vi "Add Coincident Event.vi"(8 "error in (no error)":errorcluster, 9 "Is Repeat Attempt":bool, 10 "Event":T1, 11 "Controller in":refnum<class "Controller.lvclass">) -> (0 "error out":errorcluster, 3 "Controller out":refnum<class "Controller.lvclass">)   [LabVIEW 2019, in "Controller.lvlib" / "Controller.lvclass"]
uses:
  Controller.lvclass
  <vilib>/ActorFramework/Actor/Actor.lvclass
  Controller Messages/New Event Msg/New Event Msg.lvclass
  C:/Program Files (x86)/National Instruments/LabVIEW 2019/vi.lib/ActorFramework/Actor/Actor.lvclass
  C:/Program Files (x86)/National Instruments/LabVIEW 2019/vi.lib/ActorFramework/Message/Message.lvclass
  Sensors/Detector/Event.ctl
  Sensors/Detector/Muon Detector.lvclass
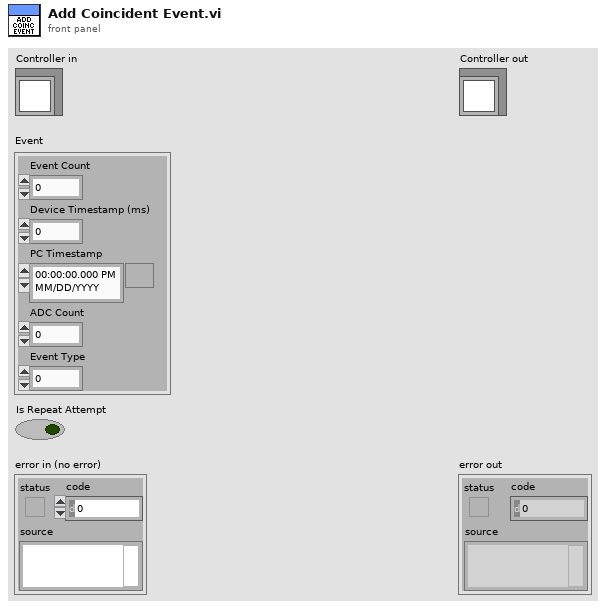
[diagram p1: front panel]
types:
  T1 = typedef "Muon Detector.lvclass/Event.ctl" = cluster{"Event Count":i32, "Device Timestamp (ms)":i32, "PC Timestamp":timestamp, "ADC Count":i32, "Event Type":u8}
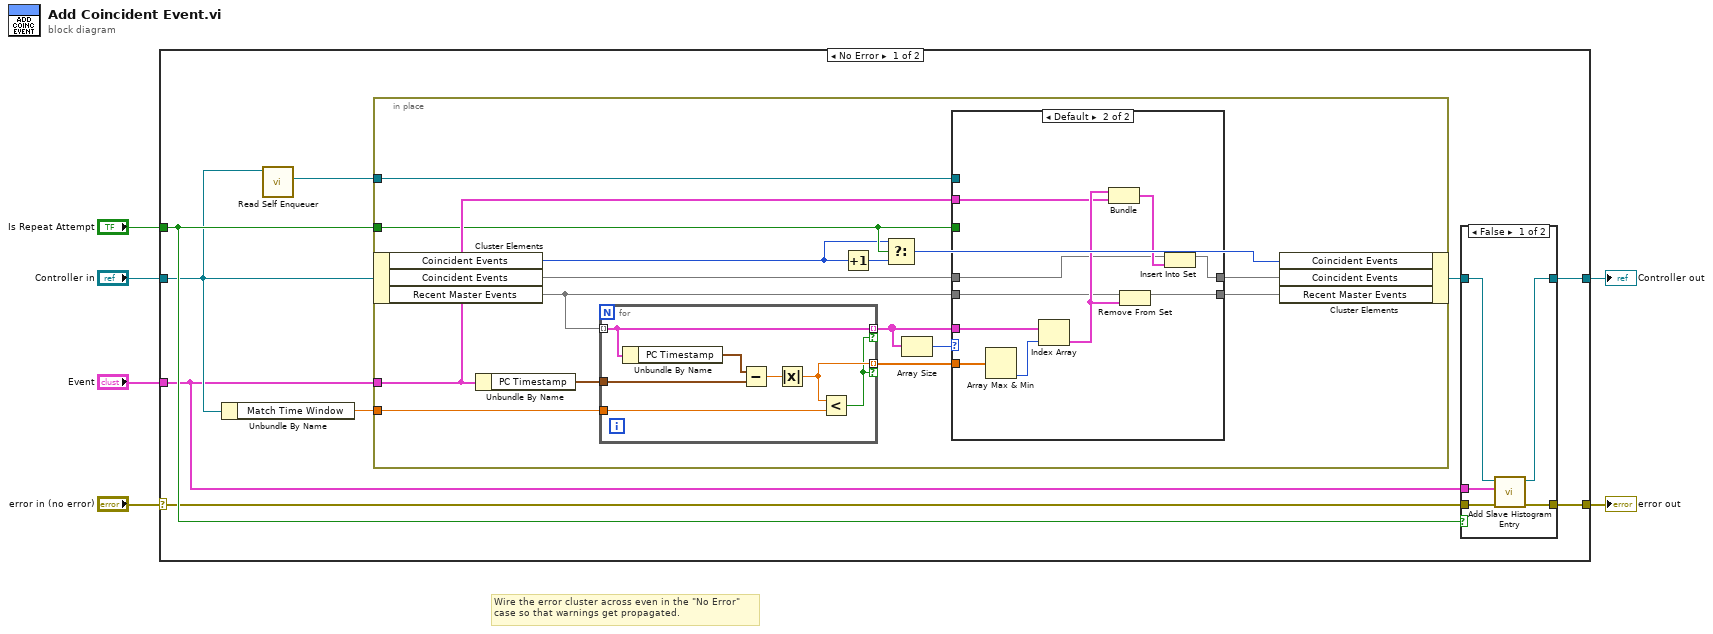
[diagram p0: block diagram]
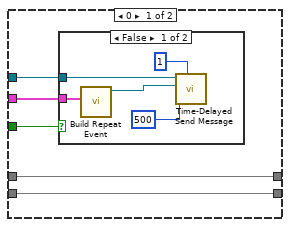
[diagram p3: hidden frame]
diagram:
  # "Wire the error cluster across even in the \"No Error\"\ncase so that warnings get propagated."
  n1 = case shown="No Error" "error in (no error)" {
    selector: "error in (no error)" -> [w13 w66]
    tunnel: [w10 w66] -> w5
    tunnel: [w8 w65] -> w3
    tunnel: "Controller in" -> [w12 w65]
    tunnel: "Event" -> [w7 _]
    tunnel: "Is Repeat Attempt" -> [w15 _]
    frame No Error {
      n2 = Unbundle By Name(w12) -> ("Match Time Window"=w14:dbl)
      n3 = call <vilib>:"Read Self Enqueuer.vi"("Actor"=w12) -> ("Self Enqueuer"=w11:refnum<class "Message Enqueuer.lvclass">)  [unwired: 10 in]
      n4 = in-place {
        in-place-border: w7 -> [w31]
        in-place-border: w14 -> [w36]
        in-place-border: w11 -> [w27]
        in-place-border: w15 -> [w26]
        n5 = in-place-cluster #1(w12) -> ("Coincident Events"=w25:i32, "Coincident Events"=w30:set{cluster{"Master":T1, "Slave":T1}}, "Recent Master Events"=w33:set{T1})
        n6 = Unbundle By Name(w31) -> ("PC Timestamp"=w37:timestamp)
        n7 = for {
          tunnel: w33 -> [w60] mode=indexing
          tunnel: w37 -> [w63]
          tunnel: w36 -> [w61]
          tunnel: [w60] -> w34 mode=indexing if=w58
          tunnel: [w59] -> w28 mode=indexing if=w58
          n8 = Unbundle By Name(w60) -> ("PC Timestamp"=w64:timestamp)
          n9 = Subtract(x=w64, y=w63) -> (x-y=w62:dbl)
          n10 = Absolute Value(x=w62) -> (abs(x)=w59:dbl)
          n11 = Less?(x=w59, y=w61) -> (x < y?=w58:bool)
        }
        n12 = Increment(x=w25) -> (x+1=w24:i32)
        n13 = Select(t=w25, s=w26, f=w24) -> (s? t:f=w23:i32)
        n14 = Array Size(array=w34) -> (size(s)=w35:i32)
        n15 = case shown="Default" w35 {
          tunnel: w34 -> [_ w55]
          tunnel: w33 -> [w42 w54]
          tunnel: [w42 w53] -> w32
          tunnel: w31 -> [w38 w52]
          tunnel: w30 -> [w41 w51]
          tunnel: [w41 w50] -> w29
          tunnel: w28 -> [_ w49]
          tunnel: w27 -> [w40 _]
          tunnel: w26 -> [w39 _]
          frame 0 {
            n16 = case shown="False" w39 {
              tunnel: w40 -> [w47 _]
              tunnel: w38 -> [w43 _]
              frame False {
                n17 = call "Build Repeat Event.vi"("Event"=w43) -> ("New Event Msg out"=w45:refnum<class "New Event Msg.lvclass">)  [unwired: 9 in, 1 out]
                n18 = call <vilib>:"Time-Delayed Send Message.vi"("# Copies (0 = infinite repeat)"=u32 1, "Milliseconds To Wait"=500, "Message"=w45, "Message Enqueuer"=w47) -> ()  [unwired: 6 in, 2 out]
              }
              frame True {
              }
            }
          }
          frame Default {
            n19 = Array Max & Min(array=w49) -> (min index (indices)=w48:i32)  [unwired: 3 out]
            n20 = Index Array(array=w55, index=w48) -> (element=w56:T1)
            n21 = Bundle("Event"=w56, "Event"=w52) -> (w57:cluster{"Event":T1, "Event":T1})  [unwired: 1 in]
            n22 = Remove From Set(10:w56, 11:w54) -> (3:w53:set{T1})  [unwired: 1 out]
            n23 = Insert Into Set(10:w57, 11:w51) -> (3:w50:set{cluster{"Master":T1, "Slave":T1}})  [unwired: 1 out]
          }
        }
        n24 = in-place-cluster #1("Coincident Events"=w23, "Coincident Events"=w29, "Recent Master Events"=w32) -> (w9:refnum<class "Controller.lvclass">)
      }
      n25 = case shown="False" w15 {
        tunnel: w13 -> [w20 w21]
        tunnel: [w19 w21] -> w10
        tunnel: w9 -> [w18 w22]
        tunnel: [w17 w22] -> w8
        tunnel: w7 -> [w16 _]
        frame False {
          n26 = call "Add Slave Histogram Entry.vi"("error in (no error)"=w20, "Event"=w16, "Controller in"=w18) -> ("error out"=w19:errorcluster, "Controller out"=w17:refnum<class "Controller.lvclass">)  [unwired: 7 in]
        }
        frame True {
        }
      }
    }
    frame Error {
    }
  }
  "error out" <- w5
  "Controller out" <- w3
